vi "Test CONNECT packet.vi"() -> ()   [LabVIEW 2013]
uses:
  Control Packets/CONNECT/CONNECT.lvclass
  Control Packets/CONNECT/ConnectFlags -- cluster.ctl
  Control Packets/ControlPacket/ControlPacket.lvclass
panel:
  out "Connect Flags":bool
  out "Keep Alive":bool
  out "Packet type":bool
  out "Client ID":bool
  out "All packets consumed":bool
  out "Complete Packet":bool
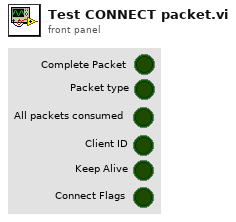
[diagram p1: front panel]
types:
  T1 = cluster{"Will Topic":string, "Will Message":string, "Username":string, "Password":string}
  T2 = typedef "CONNECT.lvclass/ConnectFlags -- cluster.ctl" = cluster{"Reserved":bool, "Clean Session":bool, "Will Flag":bool, "Will QoS 1":bool, "Will QoS 2":bool, "Will Retain":bool, "Password Flag":bool, "User Name Flag":bool}
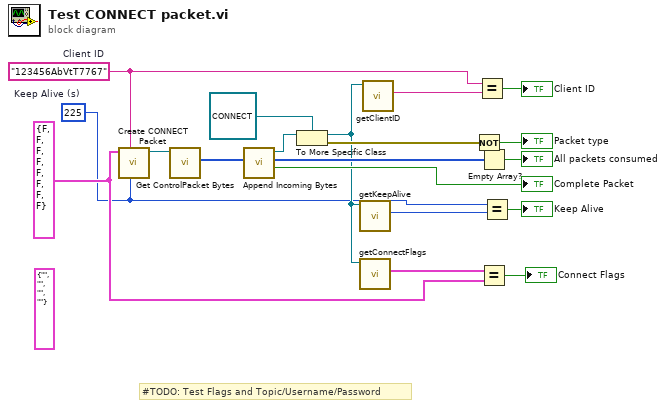
[diagram p0: block diagram]
diagram:
  (unwired) T1 {"Will Topic"="", "Will Message"="", "Username"="", "Password"=""} ("Payload")
  w2 = T2 {"Reserved"=FALSE, "Clean Session"=FALSE, "Will Flag"=FALSE, "Will QoS 1"=FALSE, "Will QoS 2"=FALSE, "Will Retain"=FALSE, "Password Flag"=FALSE, "User Name Flag"=FALSE} ("Connect Flags")
  w1 = u16 225  # Keep Alive (s)
  w14 = "123456AbVtT7767"  # Client ID
  # "#TODO: Test Flags and Topic/Username/Password"
  n1 = call "Create CONNECT Packet.vi"("Keep Alive (s)"=w1, "Client ID (empty: generate new)"=w14, "Connect Flags"=w2) -> ("CONNECT"=w19:refnum<class "CONNECT.lvclass">)  [unwired: 7 in, 1 out]
  n2 = call "Get ControlPacket Bytes.vi"("ControlPacket"=w19) -> ("Bytes Stream"=w18:u8[])  [unwired: 8 in, 2 out]
  n3 = call "Append Incoming Bytes.vi"("Incoming Packets"=w18) -> ("Complete Packet"=→"Complete Packet":bool, "Remaining Packets"=w16:u8[], "ControlPacket"=w12:refnum<class "ControlPacket.lvclass">)  [unwired: 7 in, 1 out]
  n4 = To More Specific Class(target class=refnum<class "CONNECT.lvclass"> refnum ("CONNECT in"), reference=w12) -> (specific class reference=w5:refnum<class "CONNECT.lvclass">, error out=w10:errorcluster)  [unwired: 1 in]
  n5 = call "getKeepAlive.vi"("CONNECT in"=w5) -> ("Keep Alive (s)"=w7:u16)  [unwired: 9 in, 1 out]
  n6 = call "getConnectFlags.vi"("CONNECT in"=w5) -> ("Connect Flags"=w4:T2)  [unwired: 9 in, 1 out]
  n7 = call "getClientID.vi"("CONNECT in"=w5) -> ("Client ID"=w6:string)  [unwired: 9 in, 1 out]
  n8 = Not(x=w10) -> (.not. x?=→"Packet type":bool)
  n9 = Equal?(x=w14, y=w6) -> (x = y?=→"Client ID":bool)
  n10 = Empty Array?(array=w16) -> (empty?=→"All packets consumed":bool)
  n11 = Equal?(x=w4, y=w2) -> (x = y?=→"Connect Flags":bool)
  n12 = Equal?(x=w1, y=w7) -> (x = y?=→"Keep Alive":bool)
